vi "Feed Module (Main).vi"(7 "Name of Parent Panel":string="Main.vi", 9 "New Center Coords":T1={"Horizontal"=470, "Vertical"=200}, 10 "Config":variant, 11 "Main UI Message Queue":refnum<queue>) -> ()   [LabVIEW 2018, in "Feed Module.lvlib"]
doc: "This Continuous Measurement sample project is based on the Queued Message Handler template.\n\nThe Event Handling Loop generates messages based on user interface actions.\n\nThe Message Handling Loop processes messages generated by the Event Handling Loop, or by other messages. There are also Acquisition and Logging message handling loop subVIs, and a chart updating loop."
uses:
  Feed Module.lvlib
  support/Message Queue/Message Cluster.ctl
  <vilib>/Utility/miscctls.llb/LVPoint32TypeDef.ctl
  controls/UI Data.ctl
  controls/UI State.ctl
  Controls/Feed Module Config Cluster.ctl
  Controls/Feed Module Settings Cluster.ctl
  Ismatec ISM 831C/Controls/Ismatech ISM831C Settings Cluster.ctl
  Masterflex 7550-30/Controls/Settings Cluster.ctl
  Mettler Toledo/Controls/Settings Cluster.ctl
  Bronkhorst M13 Flow Meter/Settings Cluster.ctl
  Measure Instrument/PID 2 Parameters Cluster.ctl
  Measure Instrument/PID Input Enum.ctl
  Measure Instrument/PID 2 Output Enum.ctl
  Tacmina QI/Tacmina QI DAQ Setting.ctl
  KNF Pump/Settings Cluster plus SIMDOS.ctl
  ASIA Pump/Pump Settings.ctl
  VICI M50 Party Mode/Settings Cluster.ctl
  FLOM Pump/Settings Cluster.ctl
  SSI PR Class/SSI PR or LD Settings Cluster.ctl
  Masterflex 75211/Masterflex 75211 DAQ Setting.ctl
  SSI PR Class/SSI P40 Settings Cluster.ctl
  Ismatec 78001/Ismatec 4083.ctl
  Bronkhorst M14 Flow Meter/Settings Cluster.ctl
  Controls/Feed Module State Cluster.ctl
  Controls/Feed Module Shared Variable Cluster.ctl
  Controls/Feed Module Display.ctl
  Sequencing/Squence Update Cluster.ctl
  support/Message Queue/Enqueue Message (Single).vi
  support/User Event - Stop/User Event - Stop.lvlib
  support/Support Library.lvlib
  support/Message Queue/Message Queue.lvlib
  Measure Instrument/Feed Module Engine.lvlib
  Bronkhorst M13 Flow Meter/Bronkhorst M13 Flow Meter.lvlib
  Mettler Toledo/Mettler Toledo.lvlib
  Masterflex 7550-30/Masterflex 7550-30.lvlib
  Ismatec ISM 831C/Ismatec ISM 831C.lvlib
  Operation Window.vi
  Tacmina QI/Tacmina QI.lvlib
  KNF Pump/KNF SIMDOS.lvlib
  ASIA Pump.lvlib
  Sequencing/Sequencing Library.lvlib
  VICI M50 Party Mode/VICI M6 M50 Party Mode.lvlib
  FLOM Pump/FLOM Pump.lvlib
  support/Command Log VIs/Command Logging.lvlib
  SSI PR Class/SSI PR or LD Pump.lvlib
  Masterflex 75211/Masterflex 75211.lvlib
  SSI PR Class/SSI P40 Pump.lvlib
  Ismatec 78001/Ismatec 4308.lvlib
  Bronkhorst M14 Flow Meter/Bronkhorst M14 Flow Meter.lvlib
panel:
  out "Pump On?":enum16{"Off", "On", "Not Initialized"}(ring)
  out "Pump Flow":dbl
  out "PSIG":dbl format="%#_4g"
  in  "Operation Window":bool
  out "Flow":dbl caption="g/min" format="%.2f"
  out "Ring":u16(ring)=2
  out "Log File path":path
  out "Status":string
  in  "Exit":bool
  out "kg/m^3":dbl format="%#1_4g"
  out "g":dbl format="%#_4g"
  out "C":dbl format="%#_4g"
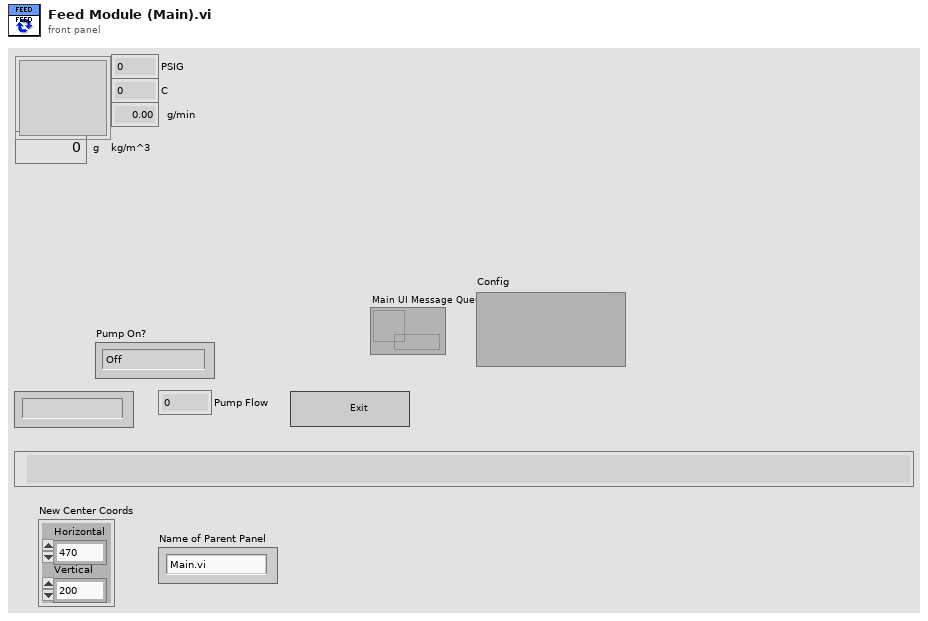
[diagram p1: front panel]
types:
  T1 = typedef "LVPoint32TypeDef.ctl" = cluster{"Horizontal":i32, "Vertical":i32}
  T2 = enum32{"Invalid", "Default", "Floating", "Floating/Auto-Hide", "Modal"}
  T3 = typedef "Feed Module.lvlib/Feed Module State Cluster.ctl" = cluster{"Shared Variables":T4, "Feed Module Config":T5}
  T4 = typedef "Feed Module.lvlib/Feed Module Shared Variable Cluster.ctl" = cluster{"PID 1 Process Variable":string, "PID 1 Output":string, "PID 1 Setpoint":string, "PID 1 Setpoint SV refnum":refnum<k21>, "PID 1 Process Variable SV refnum":refnum<k21>, "PID 1 Output SV refnum":refnum<k21>}
  T5 = typedef "Feed Module.lvlib/Feed Module Config Cluster.ctl" = cluster{"GUID":string, "Drop Coords":T1, "Process Name":string, "Queue Name":string, "Settings":T6, "Settings Load Count":i32, "OP Load Count":i32}
  T6 = typedef "Feed Module.lvlib/Feed Module Settings Cluster.ctl" = cluster{"Cycle Period":dbl, "Ismatech":T7, "Masterflex":T8, "Mettler":T9, "Bronkhorst M13 Flow Meter":T10, "PID 2 Parameters":T11, "Manual Entry":dbl, "Auto?":bool, "output range":cluster{"output high":dbl, "output low":dbl}, "Tacmina Settings":T14, "KNF SIMDOS Settings":T15, "ASIA Pump C":T16, "VICI Settings":T17, "FLOM Settings":T18, "SSI PR/LD Settings":T19, "Masterflex 75211 Settings":T20, "SSI P40 Settings":T21, "Ismatech 3 Channel Settings":T22, "Bronkhorst M14 Settings":T23}
  T7 = typedef "Ismatec ISM 831C.lvlib/Ismatech ISM831C Settings Cluster.ctl" = cluster{"VISA resource name":refnum<visa-resource-name>, "Simulated?":bool, "Pump Number":dbl, "Reverse?":bool}
  T8 = typedef "Masterflex 7550-30.lvlib/Settings Cluster.ctl" = cluster{"VISA resource name":refnum<visa-resource-name>, "Simulated?":bool, "Pump Number":dbl, "Reverse?":bool}
  T9 = typedef "Mettler Toledo.lvlib/Settings Cluster.ctl" = cluster{"VISA resource name":refnum<visa-resource-name>, "Simulated?":bool}
  T10 = typedef "Bronkhorst M13 Flow Meter.lvlib/Settings Cluster.ctl" = cluster{"VISA resource name":refnum<visa-resource-name>, "Simulated?":bool, "Smoothing Steps":i32}
  T11 = typedef "PID 2 Parameters Cluster.ctl" = cluster{"Input Device":T12, "Output Device":T13, "Setpoint":dbl, "PID gains":cluster{"proportional gain (Kc)":dbl, "integral time (Ti, min)":dbl, "derivative time (Td, min)":dbl}}
  T12 = typedef "PID Input Enum.ctl" = enum16{"Default", "Bronkhorst M13", "Bronkhorst M14", "Scale Rate of Change"}
  T13 = typedef "PID 2 Output Enum.ctl" = enum16{"Default", "Ismatec ISM 4308", "Ismatec ISM 831C", "Masterflex 7550-30", "VICI", "Tacmina QI", "KNF SIMDOS", "ASIA Type C", "FLOM UI-22-11", "SSI PR/LD", "SSI P40", "Masterflex 75211-70"}
  T14 = typedef "Tacmina QI.lvlib/Tacmina QI DAQ Setting.ctl" = cluster{"Analog DAQ Task":refnum<k21>, "Digital DAQ Task":refnum<k21>}
  T15 = typedef "KNF SIMDOS.lvlib/Settings Cluster plus SIMDOS.ctl" = cluster{"VISA resource name":refnum<visa-resource-name>, "Simulated?":bool}
  T16 = typedef "ASIA Pump.lvlib/Pump Settings.ctl" = cluster{"ASIA Pump #":i32, "channel":i32, "Simulated":bool}
  T17 = typedef "VICI M6 M50 Party Mode.lvlib/Settings Cluster.ctl" = cluster{"VISA resource name":refnum<visa-resource-name>, "Simulated?":bool, "Pump Letter":string, "Reverse?":bool}
  T18 = typedef "FLOM Pump.lvlib/Settings Cluster.ctl" = cluster{"VISA resource name":refnum<visa-resource-name>, "Simulated?":bool, "Pump Number":dbl}
  T19 = typedef "SSI PR or LD Pump.lvlib/SSI PR or LD Settings Cluster.ctl" = cluster{"VISA resource name":refnum<visa-resource-name>, "Simulated?":bool}
  T20 = typedef "Masterflex 75211.lvlib/Masterflex 75211 DAQ Setting.ctl" = cluster{"Analog DAQ Task":refnum<k21>, "Digital DAQ Task":refnum<k21>}
  T21 = typedef "SSI P40 Pump.lvlib/SSI P40 Settings Cluster.ctl" = cluster{"VISA resource name":refnum<visa-resource-name>, "Simulated?":bool}
  T22 = typedef "Ismatec 4308.lvlib/Ismatec 4083.ctl" = cluster{"VISA resource name":refnum<visa-resource-name>, "Pump Number":i16, "Channel Number":i16, "Simulated?":bool, "Reverse?":bool}
  T23 = typedef "Bronkhorst M14 Flow Meter.lvlib/Settings Cluster.ctl" = cluster{"VISA resource name":refnum<visa-resource-name>, "Simulated?":bool, "Smoothing Steps":i32}
  T24 = typedef "UI State.ctl" = enum16{"Idle", "Acquiring and Logging", "Waiting for Exit", "Waiting for Exit (Acq Stopped)", "Waiting for Exit (Log Stopped)", "Waiting for Stop", "Waiting for Stop (Acq Stopped)", "Waiting for Stop (Log Stopped)"}
  T25 = typedef "UI Data.ctl" = cluster{"Start Ref":refnum<vi>, "Trigger Ref":refnum<vi>, "Stop Ref":refnum<vi>, "Settings Ref":refnum<vi>, "Status Ref":refnum<vi>, "Exit Ref":refnum<vi>, "Data Ref":refnum<vi>}
  T26 = typedef "Feed Module.lvlib/Feed Message Queues.ctl" = cluster{"UI":refnum<queue>, "Engine":refnum<queue>, "FM Display":refnum<queue>, "OP Display":refnum<queue>}
  T27 = typedef "Feed Module.lvlib/Feed Module Display.ctl" = cluster{"Flow":dbl, "Density":dbl, "FL Temp":dbl, "Scale Value":dbl, "Pump On?":enum16{"Off", "On", "Not Initialized"}, "Cycle Period":dbl, "Input Device":T12, "Output":T13, "Pump's Pressure":dbl, "Pump's Flow ":dbl}
  T28 = cluster{"Shift":bool, "Ctrl":bool, "Alt":bool, "Cmd":bool, "Opt":bool}
  T29 = typedef "Sequencing Library.lvlib/Squence Update Cluster.ctl" = cluster{"Auto?":bool, "Manual Entry":dbl, "Setpoint":dbl}
  T30 = enum8{"Enabled", "Disabled", "Disabled and Grayed Out"}
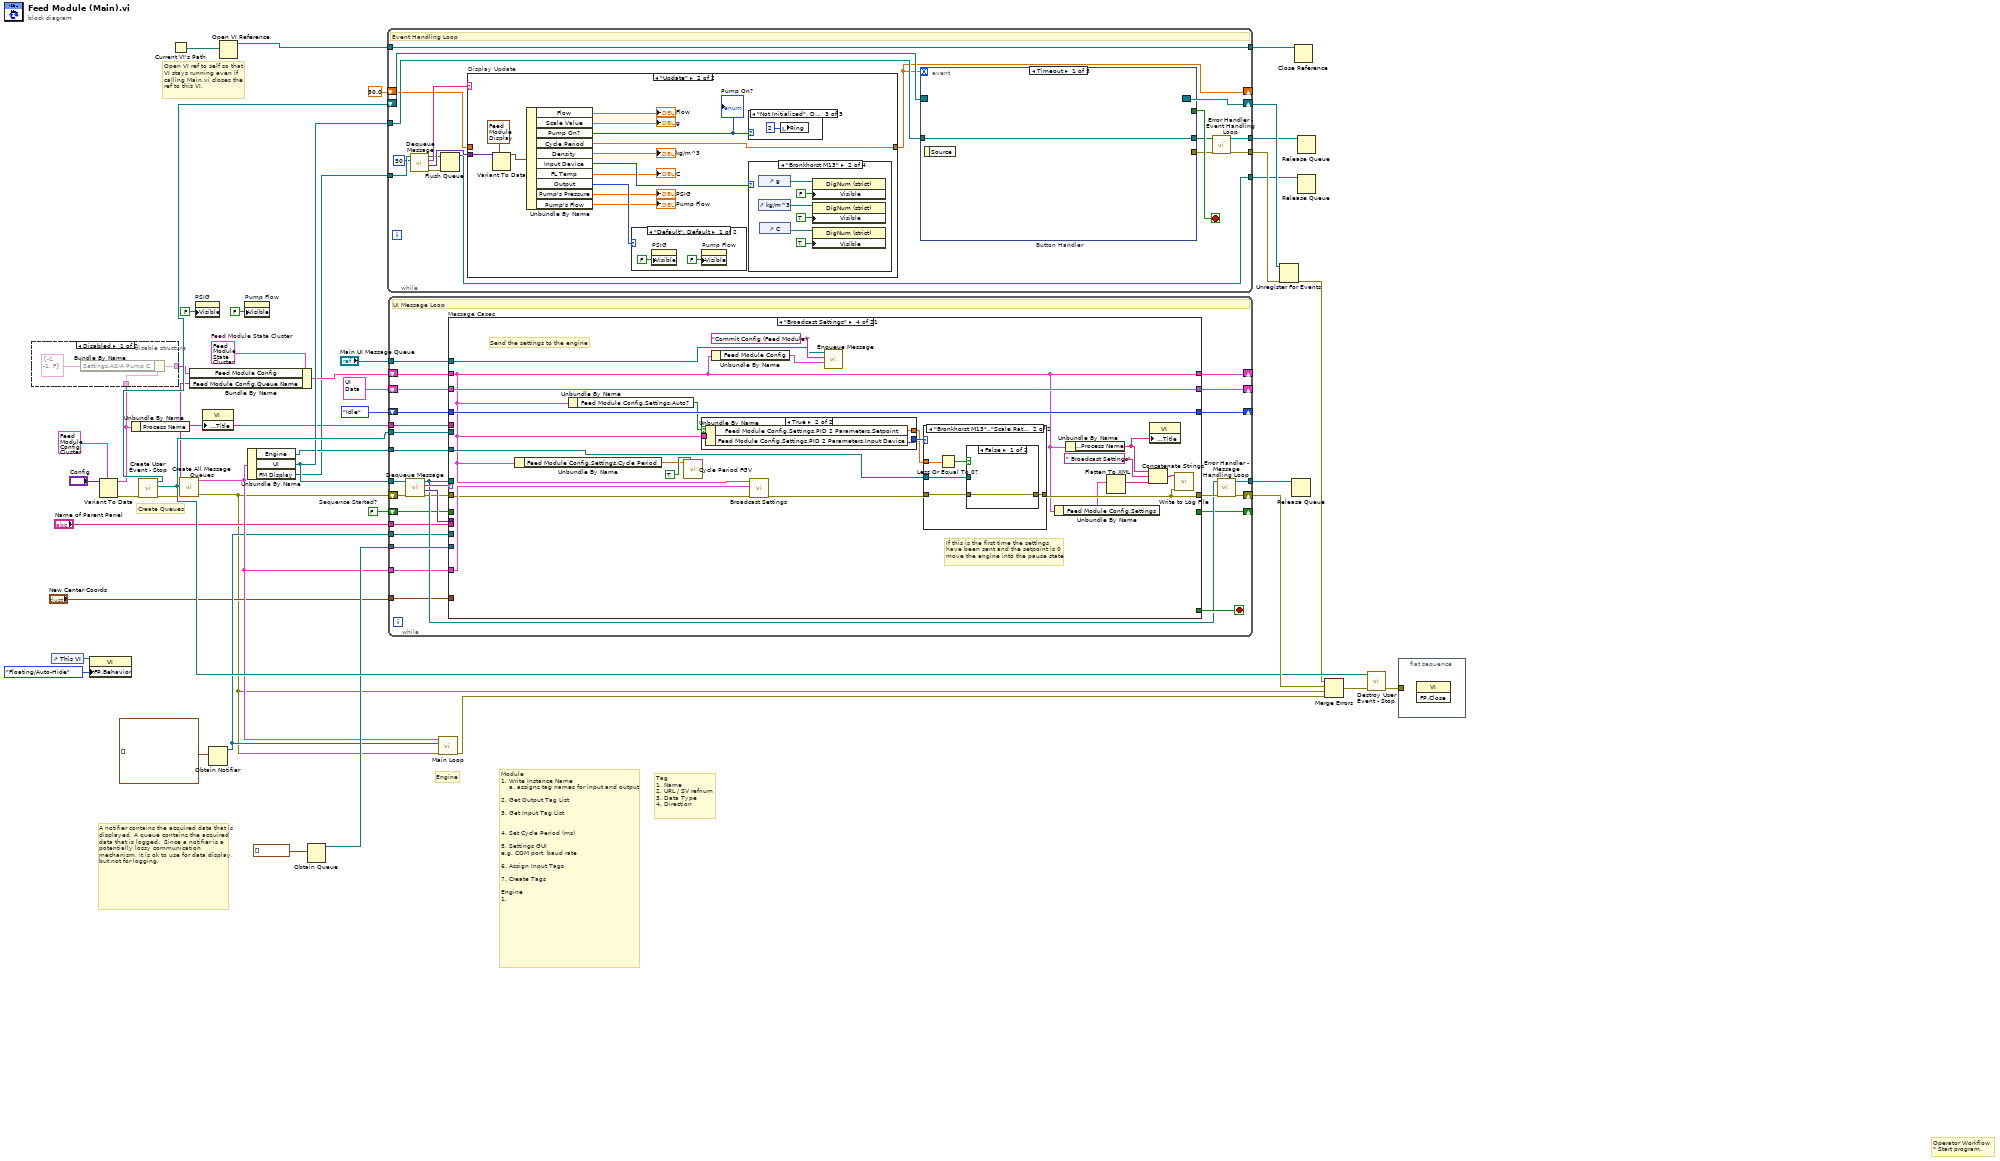
[diagram p0: block diagram]
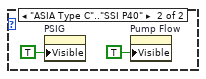
[diagram p4: hidden frame]
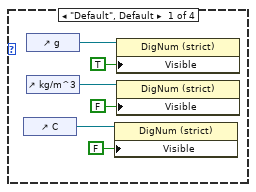
[diagram p5: hidden frame]
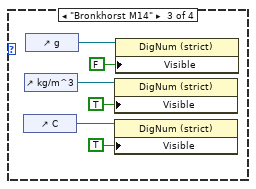
[diagram p6: hidden frame]
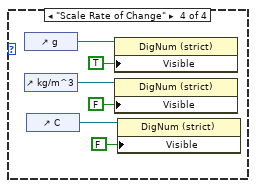
[diagram p7: hidden frame]
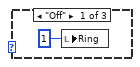
[diagram p8: hidden frame]
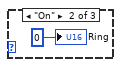
[diagram p9: hidden frame]
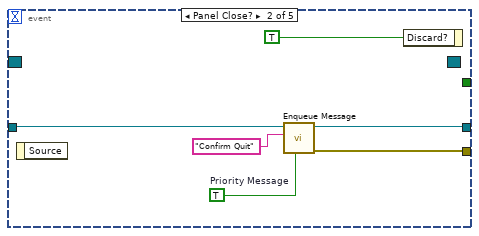
[diagram p10: hidden frame]
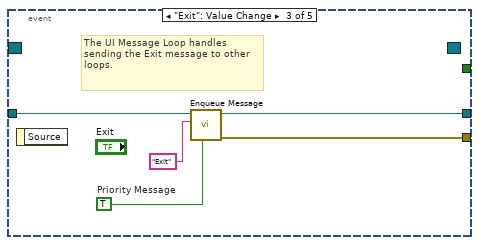
[diagram p11: hidden frame]
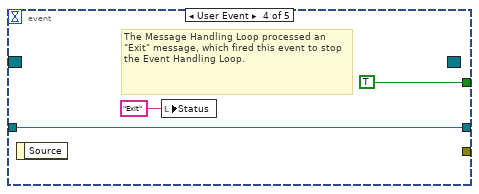
[diagram p12: hidden frame]
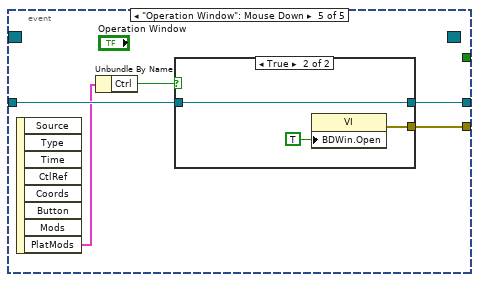
[diagram p13: hidden frame]
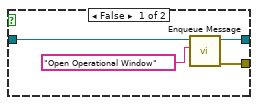
[diagram p14: hidden frame]
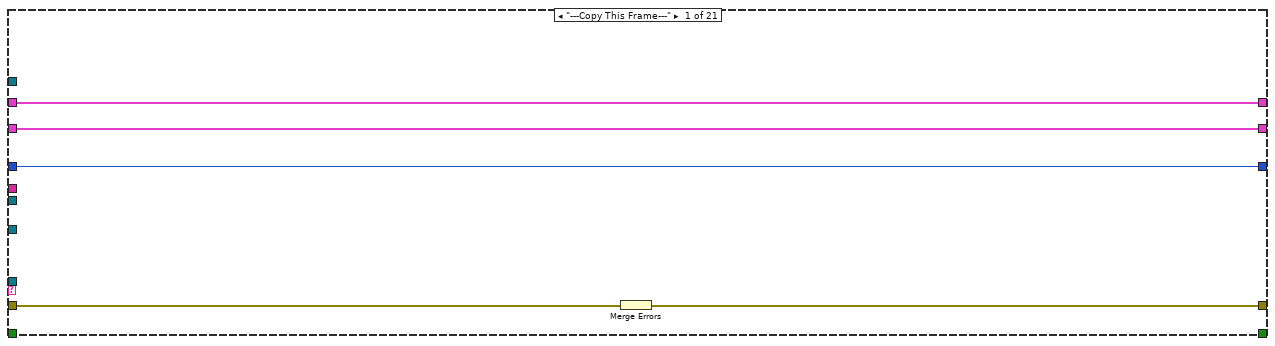
[diagram p15: hidden frame]
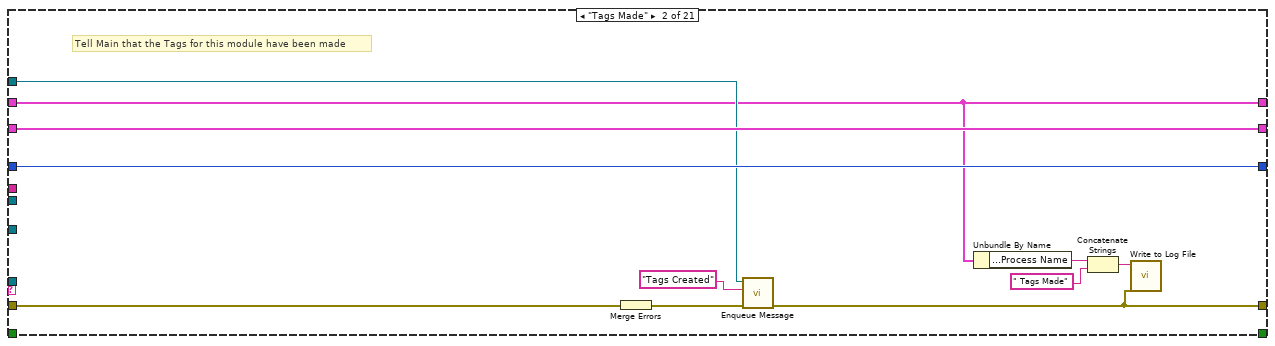
[diagram p16: hidden frame]
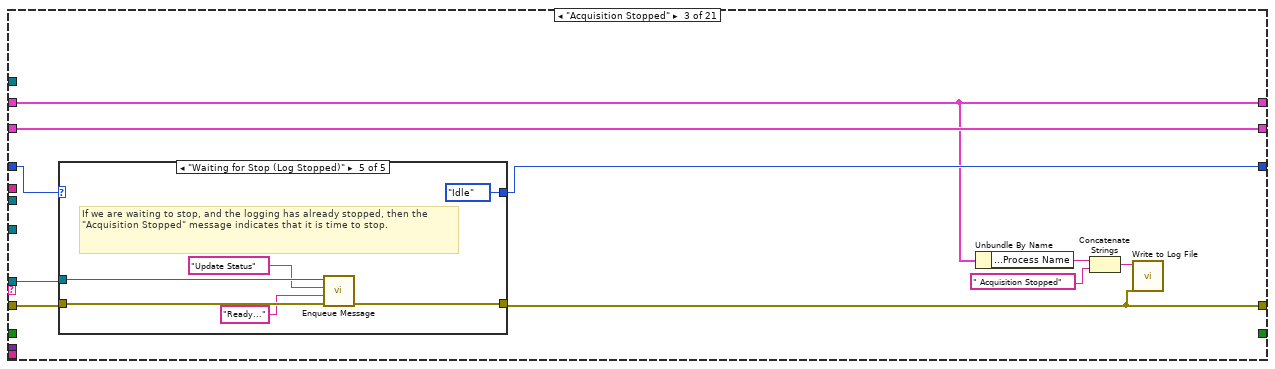
[diagram p17: hidden frame]
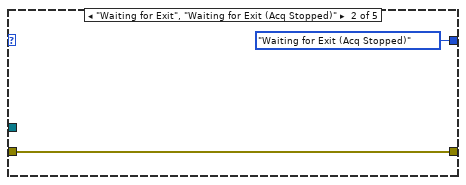
[diagram p19: hidden frame]
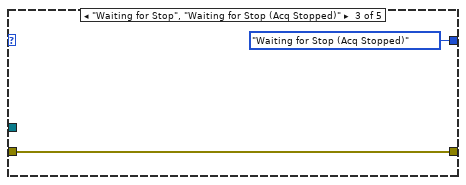
[diagram p20: hidden frame]
diagram:
  w13 = FALSE  # Sequence Started?
  w18 = T3 {"Shared Variables"={"PID 1 Process Variable"="PID1-Mettler Toledo Scale 1", "PID 1 Output"="PID1-Mettler Toledo Scale 1", "PID 1 Setpoint"="PID1-Setpoint", "PID 1 Setpoint SV refnum"="ni.var.psp://localhost/Flow Module 1/PID1-Setpoint", "PID 1 Process Variable SV refnum"="ni.var.psp://localhost/Flow Module 1/PID1-Setpoint", "PID 1 Output SV refnum"="ni.var.psp://localhost/Flow Module 1/PID1-Setpoint"}, "Feed Module Config"={"GUID"="", "Drop Coords"={"Horizontal"=0, "Vertical"=0}, "Process Name"="", "Queue Name"="", "Settings"={"Cycle Period"=500.0, "Ismatech"={"VISA resource name"="", "Simulated?"=TRUE, "Pump Number"=1.0, "Reverse?"=FALSE}, "Masterflex"={"VISA resource name"="", "Simulated?"=TRUE, "Pump Number"=1.0, "Reverse?"=FALSE}, "Mettler"={"VISA resource name"="", "Simulated?"=FALSE}, "Bronkhorst M13 Flow Meter"={"VISA resource name"="", "Simulated?"=TRUE, "Smoothing Steps"=1}, "PID 2 Parameters"={"Input Device"=enum."Default", "Output Device"=enum."Default", "Setpoint"=0.0, "PID gains"={"proportional gain (Kc)"=1.0, "integral time (Ti, min)"=0.01, "derivative time (Td, min)"=0.0}}, "Manual Entry"=0.0, "Auto?"=TRUE, "output range"={"output high"=100.0, "output low"=0.0}, "Tacmina Settings"={"Analog DAQ Task"="", "Digital DAQ Task"=""}, "KNF SIMDOS Settings"={"VISA resource name"="", "Simulated?"=TRUE}, "ASIA Pump C"={"ASIA Pump #"=0, "channel"=0, "Simulated"=FALSE}, "VICI Settings"={"VISA resource name"="", "Simulated?"=TRUE, "Pump Letter"="", "Reverse?"=FALSE}, "FLOM Settings"={"VISA resource name"="", "Simulated?"=TRUE, "Pump Number"=0.0}, "SSI PR/LD Settings"={"VISA resource name"="", "Simulated?"=FALSE}, "Masterflex 75211 Settings"={"Analog DAQ Task"="", "Digital DAQ Task"=""}, "SSI P40 Settings"={"VISA resource name"="", "Simulated?"=TRUE}, "Ismatech 3 Channel Settings"={"VISA resource name"="", "Pump Number"=1, "Channel Number"=0, "Simulated?"=TRUE, "Reverse?"=FALSE}, "Bronkhorst M14 Settings"={"VISA resource name"="", "Simulated?"=FALSE, "Smoothing Steps"=1}}, "Settings Load Count"=0, "OP Load Count"=0}}  # Feed Module State Cluster
  # "Create Queues"
  # "Open VI ref to self so that\nVI stays running even if\ncalling Main.vi closes the\nref to this VI."
  # "Engine"
  # "Operator Workflow\n* Start program."
  # "Module \n1. Write Instance Name\n    a. assigns tag names for input and output\n\n2. Get Output Tag List\n\n3. Get Input Tag List\n\n\n4. Set Cycle Period (ms)\n\n5. Settings GUI\ne.g. COM port, baud rate\n\n6. Assign Input Tags\n\n7. Create Tags\n\nEngine\n1."
  # "Tag\n1. Name\n2. URL / SV refnum\n3. Data Type\n4. Direction"
  # "A notifier contains the acquired data that is displayed. A queue contains the acquired data that is logged.  Since a notifier is a potentially lossy communication mechanism, it is ok to use for data display, but not for logging."
  n1 = control-ref of="This VI"() -> (w2:refnum<vi>)
  n2 = property class="VI"(reference=w2, "FP.Behavior"=T2."Floating/Auto-Hide" ("Front Panel Window:Behavior")) -> ()  [unwired: 1 in, 2 out]
  n3 = Variant To Data(type=T5 {"GUID"="", "Drop Coords"={"Horizontal"=0, "Vertical"=0}, "Process Name"="", "Queue Name"="", "Settings"={"Cycle Period"=500.0, "Ismatech"={"VISA resource name"="", "Simulated?"=TRUE, "Pump Number"=1.0, "Reverse?"=FALSE}, "Masterflex"={"VISA resource name"="", "Simulated?"=TRUE, "Pump Number"=1.0, "Reverse?"=FALSE}, "Mettler"={"VISA resource name"="", "Simulated?"=FALSE}, "Bronkhorst M13 Flow Meter"={"VISA resource name"="", "Simulated?"=TRUE, "Smoothing Steps"=1}, "PID 2 Parameters"={"Input Device"=enum."Default", "Output Device"=enum."Default", "Setpoint"=0.0, "PID gains"={"proportional gain (Kc)"=1.0, "integral time (Ti, min)"=0.01, "derivative time (Td, min)"=0.0}}, "Manual Entry"=0.0, "Auto?"=TRUE, "output range"={"output high"=100.0, "output low"=0.0}, "Tacmina Settings"={"Analog DAQ Task"="", "Digital DAQ Task"=""}, "KNF SIMDOS Settings"={"VISA resource name"="", "Simulated?"=TRUE}, "ASIA Pump C"={"ASIA Pump #"=0, "channel"=0, "Simulated"=FALSE}, "VICI Settings"={"VISA resource name"="", "Simulated?"=TRUE, "Pump Letter"="", "Reverse?"=FALSE}, "FLOM Settings"={"VISA resource name"="", "Simulated?"=TRUE, "Pump Number"=0.0}, "SSI PR/LD Settings"={"VISA resource name"="", "Simulated?"=FALSE}, "Masterflex 75211 Settings"={"Analog DAQ Task"="", "Digital DAQ Task"=""}, "SSI P40 Settings"={"VISA resource name"="", "Simulated?"=TRUE}, "Ismatech 3 Channel Settings"={"VISA resource name"="", "Pump Number"=1, "Channel Number"=0, "Simulated?"=TRUE, "Reverse?"=FALSE}, "Bronkhorst M14 Settings"={"VISA resource name"="", "Simulated?"=FALSE, "Smoothing Steps"=1}}, "Settings Load Count"=0, "OP Load Count"=0} ("Feed Module Config"), Variant="Config") -> (data=w9:T5, error out=w21:errorcluster)  [unwired: 1 in]
  n4 = disable-structure shown="Disabled" {
    disable-tunnel: w9 -> [w46 w48]
    disable-tunnel: [w45 w48] -> w8
    frame Disabled {
      n5 = Bundle By Name(cluster=w46, "Settings.ASIA Pump C"=T16 {"ASIA Pump #"=-1, "channel"=-1, "Simulated"=FALSE}) -> (w45:T5)
    }
    frame Enabled {
    }
  }
  n6 = Unbundle By Name(w9) -> ("Process Name"=w7:string)
  n7 = call "Create User Event - Stop.vi"("error in (no error)"=w21) -> ("error out"=w39:errorcluster, "User Event - Stop"=w40:refnum<user-event>, "Stop Event Registration Refnum"=w41:refnum<event-registration>)  [unwired: 8 in]
  n8 = Current VI's Path() -> (path=w24:path)
  n9 = call "Create All Message Queues.vi"("error in (no error)"=w39, "Process Name"=w7) -> ("error out"=w12:errorcluster, "Message Queues"=w28:T26)  [unwired: 8 in]
  n10 = Bundle By Name(cluster=w18, "Feed Module Config"=w8, "Feed Module Config.Queue Name"=w7) -> (w22:T3)
  n11 = property on="PSIG" class="DigNum (strict)"("Visible"=FALSE) -> ()  [unwired: 2 in, 2 out]
  n12 = property class="VI"("Front Panel.Title"=w7) -> ()  [unwired: 2 in, 2 out]
  n13 = Obtain Notifier(notification data type=waveform(dbl)[] []) -> (notifier out=w27:refnum<notifier>)  [unwired: 3 in, 2 out]
  n14 = Open VI Reference(vi path=w24) -> (vi reference=w25:refnum<vi>)  [unwired: 5 in, 1 out]
  n15 = property on="Pump Flow" class="DigNum (strict)"("Visible"=FALSE) -> ()  [unwired: 2 in, 2 out]
  n16 = Unbundle By Name(w28) -> ("Engine"=w31:refnum<queue>, "UI"=w35:refnum<queue>, "FM Display"=w17:refnum<queue>)
  n17 = Obtain Queue(element data type=waveform(dbl)[] []) -> (queue out=w30:refnum<queue>)  [unwired: 4 in, 2 out]
  n18 = while {
    tunnel: w35 -> [w60]
    tunnel: [w62] -> w43
    shift-right: [w61] -> w37
    shift-left: w41 -> [w66]
    tunnel: [w59] -> w26
    tunnel: w25 -> [w59]
    tunnel: w17 -> [w58]
    shift-right: [w55] -> _
    shift-left: 50.0 ("Cycle Period") -> [w54]
    tunnel: [w50] -> w5
    tunnel: [w49] -> w4
    stop <- w65 stop-if-true
    # "Event Handling Loop"
    n19 = call "Dequeue Message.vi"("timeout in ms (-1)"=50, "Message Queue"=w58) -> ("error out"=w51:errorcluster, "Message Data"=w56:variant, "Message"=w57:string, "dup Message Queue"=w52:refnum<queue>)  [unwired: 6 in]
    n20 = Flush Queue(queue=w52, error in (no error)=w51) -> (queue out=w49:refnum<queue>)  [unwired: 2 out]
    n21 = case "Display Update" shown="\"Update\"" w57 {
      tunnel: w56 -> [_ w80]
      tunnel: [w67 w74] -> w55
      tunnel: w54 -> [w67 _]
      frame "False", Default {
      }
      frame "Update" {
        n22 = Variant To Data(type=T27 {"Flow"=0.0, "Density"=0.0, "FL Temp"=0.0, "Scale Value"=0.0, "Pump On?"=enum."Off", "Cycle Period"=500.0, "Input Device"=enum."Bronkhorst M13", "Output"=enum."Default", "Pump's Pressure"=0.0, "Pump's Flow "=0.0}, Variant=w80) -> (data=w78:T27)  [unwired: 1 in, 1 out]
        n23 = Unbundle By Name(w78) -> ("Flow"=→"Flow":dbl, "Scale Value"=→"g":dbl, "Pump On?"=w75:enum16{"Off", "On", "Not Initialized"}, "Cycle Period"=w74:dbl, "Density"=→"kg/m^3":dbl, "Input Device"=w73:T12, "FL Temp"=→"C":dbl, "Output"=w70:T13, "Pump's Pressure"=→"PSIG":dbl, "Pump's Flow"=→"Pump Flow":dbl)
        "Pump On?" <- w75
        n24 = case shown="\"Default\", Default" w70 {
          frame "Default", Default {
            n25 = property on="PSIG" class="DigNum (strict)"("Visible"=FALSE) -> ()  [unwired: 2 in, 2 out]
            n26 = property on="Pump Flow" class="DigNum (strict)"("Visible"=FALSE) -> ()  [unwired: 2 in, 2 out]
          }
          frame "ASIA Type C".."SSI P40" {
            n27 = property on="PSIG" class="DigNum (strict)"("Visible"=TRUE) -> ()  [unwired: 2 in, 2 out]
            n28 = property on="Pump Flow" class="DigNum (strict)"("Visible"=TRUE) -> ()  [unwired: 2 in, 2 out]
          }
        }
        n29 = case shown="\"Not Initialized\", Default" w75 {
          frame "Off" {
            n30 = local write "Ring"(u16 1 ("Ring")) -> ()
          }
          frame "On" {
            "Ring" <- u16 0 ("Ring")
          }
          frame "Not Initialized", Default {
            n31 = local write "Ring"(u16 2 ("Ring")) -> ()
          }
        }
        n32 = case shown="\"Bronkhorst M13\"" w73 {
          frame "Default", Default {
            n33 = control-ref of="C"() -> (w86:refnum<vi>)
            n34 = control-ref of="g"() -> (w89:refnum<vi>)
            n35 = control-ref of="kg/m^3"() -> (w90:refnum<vi>)
            n36 = property class="DigNum (strict)"(reference=w86, "Visible"=FALSE) -> ()  [unwired: 1 in, 2 out]
            n37 = property class="DigNum (strict)"(reference=w89, "Visible"=TRUE) -> ()  [unwired: 1 in, 2 out]
            n38 = property class="DigNum (strict)"(reference=w90, "Visible"=FALSE) -> ()  [unwired: 1 in, 2 out]
          }
          frame "Bronkhorst M13" {
            n39 = control-ref of="g"() -> (w95:refnum<vi>)
            n40 = control-ref of="kg/m^3"() -> (w96:refnum<vi>)
            n41 = control-ref of="C"() -> (w92:refnum<vi>)
            n42 = property class="DigNum (strict)"(reference=w95, "Visible"=FALSE) -> ()  [unwired: 1 in, 2 out]
            n43 = property class="DigNum (strict)"(reference=w96, "Visible"=TRUE) -> ()  [unwired: 1 in, 2 out]
            n44 = property class="DigNum (strict)"(reference=w92, "Visible"=TRUE) -> ()  [unwired: 1 in, 2 out]
          }
          frame "Bronkhorst M14" {
            n45 = control-ref of="C"() -> (w97:refnum<vi>)
            n46 = control-ref of="kg/m^3"() -> (w102:refnum<vi>)
            n47 = control-ref of="g"() -> (w101:refnum<vi>)
            n48 = property class="DigNum (strict)"(reference=w102, "Visible"=TRUE) -> ()  [unwired: 1 in, 2 out]
            n49 = property class="DigNum (strict)"(reference=w97, "Visible"=TRUE) -> ()  [unwired: 1 in, 2 out]
            n50 = property class="DigNum (strict)"(reference=w101, "Visible"=FALSE) -> ()  [unwired: 1 in, 2 out]
          }
          frame "Scale Rate of Change" {
            n51 = control-ref of="g"() -> (w107:refnum<vi>)
            n52 = control-ref of="kg/m^3"() -> (w108:refnum<vi>)
            n53 = control-ref of="C"() -> (w103:refnum<vi>)
            n54 = property class="DigNum (strict)"(reference=w107, "Visible"=TRUE) -> ()  [unwired: 1 in, 2 out]
            n55 = property class="DigNum (strict)"(reference=w108, "Visible"=FALSE) -> ()  [unwired: 1 in, 2 out]
            n56 = property class="DigNum (strict)"(reference=w103, "Visible"=FALSE) -> ()  [unwired: 1 in, 2 out]
          }
        }
      }
    }
    n57 = event "Button Handler" shown="[0] Timeout" {
      selector: w66 -> [_ _ _ _ _]
      dyn-events: [_ _ _ _ _] -> w61
      timeout: w55 -> [_ _ _ _ _]
      tunnel: [_ _ _ TRUE ("Discard?") _] -> w65
      tunnel: w60 -> [w112 w115 w120 w124 w129]
      tunnel: [_ w113 w123 _ w131] -> w63
      tunnel: [w112 w114 w119 w124 w130] -> w64
      event Timeout {
        n58 = event-data() -> ()  [unwired: 1 in, 1 out]
      }
      event Panel Close? {
        w116 = TRUE  # Priority Message
        n59 = event-data() -> ()  [unwired: 1 in, 1 out]
        n60 = call-poly "Enqueue Message.vi"("Priority Message? (F)"=w116, "Message"="Confirm Quit", "Message Queue"=w115) -> ("error out"=w113:errorcluster, "dup Message Queue"=w114:refnum<queue>)  [unwired: 7 in]
        n61 = event-data("Discard?"=TRUE) -> ()  [unwired: 1 in, 1 out]
      }
      event "Exit": Value Change {
        w121 = TRUE  # Priority Message
        # "The UI Message Loop handles sending the Exit message to other loops."
        n62 = event-data() -> ()  [unwired: 1 in, 1 out]
        n63 = call-poly "Enqueue Message.vi"("Priority Message? (F)"=w121, "Message"="Exit", "Message Queue"=w120) -> ("error out"=w123:errorcluster, "dup Message Queue"=w119:refnum<queue>)  [unwired: 7 in]
      }
      event User Event {
        # "The Message Handling Loop processed an \"Exit\" message, which fired this event to stop the Event Handling Loop."
        n64 = event-data() -> ()  [unwired: 1 in, 1 out]
        n65 = local write "Status"("Exit" ("Exit String")) -> ()
      }
      event "Operation Window": Mouse Down {
        n66 = event-data() -> ("PlatMods"=w128:T28)  [unwired: 1 in, 7 out]
        n67 = Unbundle By Name(w128) -> ("Ctrl"=w127:bool)
        n68 = case shown="True" w127 {
          tunnel: [w135 w136] -> w131
          tunnel: [w134 w137] -> w130
          tunnel: w129 -> [w133 w137]
          frame False {
            n69 = call-poly "Enqueue Message.vi"("Message"="Open Operational Window", "Message Queue"=w133) -> ("error out"=w135:errorcluster, "dup Message Queue"=w134:refnum<queue>)  [unwired: 8 in]
          }
          frame True {
            n70 = property class="VI"("BDWin.Open"=TRUE ("Block Diagram Window:Open")) -> (error out=w136:errorcluster)  [unwired: 2 in, 1 out]
          }
        }
      }
    }
    n71 = call "Error Handler - Event Handling Loop.vi"("error in (no error)"=w63, "Message Queue"=w64) -> ("dup error in"=w62:errorcluster, "dup Message Queue"=w50:refnum<queue>)  [unwired: 8 in]
  }
  n72 = while {
    tunnel: w35 -> [w160]
    tunnel: w40 -> [w164]
    shift-right: [w154] -> w44
    shift-left: w12 -> [w163]
    shift-right: [w159] -> _
    shift-left: w22 -> [w142]
    shift-right: [w157] -> _
    shift-left: T25 {"Start Ref"=refnum, "Trigger Ref"=refnum, "Stop Ref"=refnum, "Settings Ref"=refnum, "Status Ref"=refnum, "Exit Ref"=refnum, "Data Ref"=refnum} ("Measurement UI Controls") -> [w158]
    tunnel: w27 -> [w144]
    tunnel: w30 -> [w156]
    shift-right: [w152] -> _
    shift-left: UI_State."Idle" ("UI State") -> [w146]
    tunnel: w31 -> [w151]
    tunnel: w28 -> [w143]
    tunnel: "Main UI Message Queue" -> [w147]
    tunnel: "Name of Parent Panel" -> [w150]
    tunnel: w7 -> [w149]
    tunnel: "New Center Coords" -> [w148]
    shift-right: [w140] -> _
    shift-left: w13 -> [w141]
    tunnel: [w139] -> w3
    stop <- w165 stop-if-true
    # "UI Message Loop"
    n73 = call "Dequeue Message.vi"("error in (no error)"=w163, "Message Queue"=w160) -> ("error out"=w145:errorcluster, "Message Data"=w161:variant, "Message"=w162:string, "dup Message Queue"=w153:refnum<queue>)  [unwired: 6 in]
    n74 = case "Message Cases" shown="\"Broadcast Settings\"" w162 {
      selector: w162 -> [_ _ _ _ _ _ _ _ _ _ _ _ _ _ _ _ _ _ _ _ w595]
      tunnel: w153 -> [_ _ w187 _ w255 _ w311 w327 w358 w383 _ w421 w439 w453 _ w501 _ _ w572 _ _]
      tunnel: w145 -> [w170 w181 w188 w225 w254 w280 w296 w326 w362 w387 w406 w416 _ w454 w485 w499 w518 w532 w557 w589 _]
      tunnel: [w169 w172 w183 w217 w249 w281 w288 w315 w347 w365 w406 w408 w431 w449 w481 w493 w520 w534 w549 w576 w596] -> w155
      tunnel: [_ _ _ _ _ _ _ _ _ TRUE _ _ _ _ _ _ _ _ _ _ _] -> w165
      tunnel: w161 -> [_ _ _ _ _ w283 _ _ w361 w371 _ _ w437 _ _ _ _ _ _ w588 _]
      tunnel: w164 -> [_ _ _ _ _ _ _ _ _ w386 _ _ _ _ _ _ _ _ _ _ _]
      tunnel: [w168 w171 w182 w211 w248 w286 w287 w314 w349 w364 w405 w407 w429 w448 w480 w492 w519 w533 w548 w575 w601] -> w159
      tunnel: w158 -> [w167 w180 w191 w230 w257 w285 w308 w324 w363 w384 w404 w417 w441 w457 w489 w516 w525 w542 w569 w585 w606]
      tunnel: [w167 w180 w191 w230 w257 w285 w308 w324 w363 w384 w403 w417 w441 w457 w489 w516 w525 w542 w569 w585 w606] -> w157
      tunnel: w156 -> [_ _ _ _ _ _ _ _ _ w378 _ _ _ _ _ _ _ _ _ _ _]
      tunnel: w146 -> [w166 w179 w190 w229 w256 w279 w297 _ w353 _ _ _ w440 w456 w477 _ _ _ w558 w580 w605]
      tunnel: [w166 w179 w189 w229 w253 w279 w298 UI_State."Acquiring and Logging" ("UI State") w353 UI_State."Idle" ("UI State") UI_State."Idle" ("UI State") UI_State."Idle" ("UI State") w440 w455 w477 UI_State."Acquiring and Logging" ("UI State") UI_State."Acquiring and Logging" ("UI State") UI_State."Acquiring and Logging" ("UI State") w559 w580 w605] -> w152
      tunnel: w151 -> [_ _ _ w224 _ _ w295 _ _ w376 _ _ _ _ _ _ w523 w540 w556 _ _]
      tunnel: w150 -> [_ _ _ _ _ _ _ _ _ _ _ w415 _ _ _ _ _ _ _ _ _]
      tunnel: w149 -> [_ _ _ _ _ _ _ _ _ _ _ w412 _ _ _ _ _ _ _ _ _]
      tunnel: w148 -> [_ _ _ _ _ _ _ _ _ _ _ w414 _ _ _ _ _ _ _ _ _]
      tunnel: w147 -> [_ w177 _ w210 _ _ _ _ _ w369 _ _ _ _ w488 _ _ _ _ _ _]
      tunnel: w144 -> [_ _ _ _ _ _ _ _ _ w382 _ _ _ _ w487 _ _ _ _ _ _]
      tunnel: w143 -> [_ _ _ w228 _ _ _ _ _ _ _ _ _ _ w486 _ _ _ _ _ _]
      tunnel: w142 -> [w168 w171 w182 w211 w248 w286 w287 w314 w349 w364 w405 w407 w430 w448 w479 w492 w519 w533 w548 w575 w601]
      tunnel: w141 -> [_ _ _ _ _ _ _ w323 _ _ _ _ _ _ _ _ _ _ _ _ _]
      tunnel: [_ _ _ _ _ _ _ w320 _ _ _ _ _ _ _ _ _ _ _ _ _] -> w140
      frame "---Copy This Frame---" {
        # "Duplicate this frame when creating new messages.  Change this comment in the duplicated frame to describe this message."
        n75 = Merge Errors(w170) -> (w169:errorcluster)
      }
      frame "Tags Made" {
        # "Tell Main that the Tags for this module have been made"
        # "Duplicate this frame when creating new messages.  Change this comment in the duplicated frame to describe this message."
        n76 = Merge Errors(w181) -> (w176:errorcluster)
        n77 = call-poly "Enqueue Message.vi"("error in (no error)"=w176, "Message"="Tags Created", "Message Queue"=w177) -> ("error out"=w172:errorcluster)  [unwired: 7 in, 1 out]
        n78 = Unbundle By Name(w171) -> ("Feed Module Config.Process Name"=w175:string)
        n79 = Concatenate Strings(w175, " Tags Made" ("text")) -> (w173:string)
        n80 = call "Write to Log File.vi"("error in"=w172, "text"=w173) -> ()  [unwired: 9 in, 1 out]
      }
      frame "Acquisition Stopped" {
        # "Logic for determining what action to take when the acquisition has stopped."
        n81 = case shown="\"Waiting for Stop (Log Stopped)\"" w190 {
          selector: w190 -> [w193 _ _ _ _]
          tunnel: [w193 UI_State."Waiting for Exit (Acq Stopped)" ("UI State") UI_State."Waiting for Stop (Acq Stopped)" ("UI State") UI_State."Idle" ("UI State") UI_State."Idle" ("UI State")] -> w189
          tunnel: w188 -> [w192 w194 w196 w202 w208]
          tunnel: [w192 w194 w196 w201 w207] -> w183
          tunnel: w187 -> [_ _ _ w200 w206]
          frame Default {
          }
          frame "Waiting for Exit", "Waiting for Exit (Acq Stopped)" {
          }
          frame "Waiting for Stop", "Waiting for Stop (Acq Stopped)" {
          }
          frame "Waiting for Exit (Log Stopped)" {
            # "If we are waiting to exit, and the logging has already stopped, then the \"Acquisition Stopped\" message indicates that it is time to exit."
            n82 = call-poly "Enqueue Message.vi"("Priority Message? (F)"=TRUE, "error in (no error)"=w202, "Message"="Exit", "Message Queue"=w200) -> ("error out"=w201:errorcluster)  [unwired: 6 in, 1 out]
          }
          frame "Waiting for Stop (Log Stopped)" {
            # "If we are waiting to stop, and the logging has already stopped, then the \"Acquisition Stopped\" message indicates that it is time to stop."
            n83 = call-poly "Enqueue Message.vi"("error in (no error)"=w208, "Message Data"="Ready..." ("Message"), "Message"="Update Status", "Message Queue"=w206) -> ("error out"=w207:errorcluster)  [unwired: 6 in, 1 out]
          }
        }
        n84 = Unbundle By Name(w182) -> ("Feed Module Config.Process Name"=w186:string)
        n85 = Concatenate Strings(w186, " Acquisition Stopped" ("text")) -> (w184:string)
        n86 = call "Write to Log File.vi"("error in"=w183, "text"=w184) -> ()  [unwired: 9 in, 1 out]
      }
      frame "Broadcast Settings" {
        # "If this is the first time the settings\nhave been sent and the setpoint is 0 \nmove the engine into the pause state"
        # "Send the settings to the engine"
        # "Send the 'Update Settings' message to the Logging and Acquisition message loops."
        n87 = Unbundle By Name(w211) -> ("Feed Module Config.Settings.Cycle Period"=w226:dbl)
        n88 = Unbundle By Name(w211) -> ("Feed Module Config.Settings.Auto?"=w220:bool)
        n89 = call "Cycle Period FGV.vi"("Write"=TRUE, "Cycle Period In (ms)"=w226) -> ()  [unwired: 8 in, 2 out]
        n90 = case shown="True" w220 {
          tunnel: [w231 w236] -> w222
          tunnel: [w232 w235] -> w221
          tunnel: w211 -> [w233 w234]
          frame False {
            n91 = Unbundle By Name(w233) -> ("Feed Module Config.Settings.Manual Entry"=w232:dbl, "Feed Module Config.Settings.PID 2 Parameters.Input Device"=w231:T12)
          }
          frame True {
            n92 = Unbundle By Name(w234) -> ("Feed Module Config.Settings.PID 2 Parameters.Setpoint"=w235:dbl, "Feed Module Config.Settings.PID 2 Parameters.Input Device"=w236:T12)
          }
        }
        n93 = Unbundle By Name(w211) -> ("Feed Module Config"=w213:T5)
        n94 = call "Broadcast Settings.vi"("error in (no error)"=w225, "Message Queues"=w228, "Feed Module State Cluster in"=w211) -> ("error out"=w223:errorcluster)  [unwired: 8 in]
        n95 = call-poly "Enqueue Message.vi"("Message Data"=w213, "Message"="Commit Config (Feed Module)", "Message Queue"=w210) -> ()  [unwired: 7 in, 2 out]
        n96 = case shown="\"Bronkhorst M13\"..\"Scale Rate of Change\"" w222 {
          tunnel: w223 -> [w237 w242]
          tunnel: w224 -> [_ w241]
          tunnel: [w237 w240] -> w217
          tunnel: w221 -> [_ w239]
          frame "Default", Default {
          }
          frame "Bronkhorst M13".."Scale Rate of Change" {
            n97 = Less Or Equal To 0?(x=w239) -> (x <= 0?=w238:bool)
            n98 = case shown="False" w238 {
              tunnel: w242 -> [w243 w247]
              tunnel: w241 -> [_ w246]
              tunnel: [w243 w245] -> w240
              frame False {
              }
              frame True {
                n99 = call-poly "Enqueue Message.vi"("error in (no error)"=w247, "Message"="Pause", "Message Queue"=w246) -> ("error out"=w245:errorcluster)  [unwired: 7 in, 1 out]
              }
            }
          }
        }
        n100 = Unbundle By Name(w211) -> ("Feed Module Config.Settings"=w216:T6)
        n101 = Unbundle By Name(w211) -> ("Feed Module Config.Process Name"=w214:string)
        n102 = Flatten To XML(anything=w216) -> (xml string=w215:string)
        n103 = Concatenate Strings(w214, " Broadcast Settings" ("text"), w215) -> (w218:string)
        n104 = property class="VI"("Front Panel.Title"=w214) -> ()  [unwired: 2 in, 2 out]
        n105 = call "Write to Log File.vi"("error in"=w217, "text"=w218) -> ()  [unwired: 9 in, 1 out]
      }
      frame "Confirm Quit" {
        # "Confirm Quit - Message that can confirm whether or not the user wants to exit the application."
        n106 = case shown="\"Acquiring and Logging\"" w256 {
          tunnel: w255 -> [w262 w268]
          tunnel: w254 -> [w261 w266]
          tunnel: [w258 w265] -> w249
          tunnel: [UI_State."Idle" ("UI State") w264] -> w253
          frame Default {
            # "If 'Confirm Quit' comes in while the system is idle, there is no need for a confirmation message."
            n107 = call-poly "Enqueue Message.vi"("Priority Message? (F)"=TRUE, "error in (no error)"=w261, "Message"="Exit", "Message Queue"=w262) -> ("error out"=w258:errorcluster)  [unwired: 6 in, 1 out]
          }
          frame "Acquiring and Logging" {
            n108 = Two Button Dialog(message="Are you sure you want to quit while the acquisition is running?" ("Confirm Quit Message"), 1:"No" ("No"), 2:"Yes" ("Yes")) -> (T button?=w267:bool)
            n109 = case shown="True" w267 {
              tunnel: w268 -> [_ w278]
              tunnel: w266 -> [w272 w277]
              tunnel: [w272 w276] -> w265
              tunnel: [UI_State."Acquiring and Logging" ("UI State") UI_State."Waiting for Exit" ("UI State")] -> w264
              frame False {
                # "User did not want to quit."
              }
              frame True {
                n110 = call-poly "Enqueue Message.vi"("error in (no error)"=w277, "Message"="Stop", "Message Queue"=w278) -> ("error out"=w276:errorcluster)  [unwired: 7 in, 1 out]
              }
            }
          }
        }
        n111 = Unbundle By Name(w248) -> ("Feed Module Config.Process Name"=w252:string)
        n112 = Concatenate Strings(w252, " Quit" ("text")) -> (w250:string)
        n113 = call "Write to Log File.vi"("error in"=w249, "text"=w250) -> ()  [unwired: 9 in, 1 out]
      }
      frame "Display Log File Path" {
        n114 = Variant To Data(error in=w280, type=path "", Variant=w283) -> (data=→"Log File path":path, error out=w281:errorcluster)
      }
      frame "E-Stop" {
        # "E-Stop pauses the engine"
        # "Message Acquisition and Logging loops to stop"
        # "Enable: Start, Exit, Settings\nDisable: Stop"
        # "Stop the pumps."
        n115 = Unbundle By Name(w308) -> ("Trigger Ref"=w299:refnum<vi>, "Stop Ref"=w300:refnum<vi>, "Start Ref"=w303:refnum<vi>, "Exit Ref"=w302:refnum<vi>, "Settings Ref"=w301:refnum<vi>)
        n116 = call-poly "Enqueue Message.vi"("error in (no error)"=w296, "Message Data"="Ready..." ("Ready..."), "Message"="Update Status", "Message Queue"=w311) -> ("error out"=w293:errorcluster)  [unwired: 6 in, 1 out]
        n117 = Build Array(w303, w302, w301) -> (w306:refnum<vi>[])
        n118 = Build Array(w299, w300) -> (w305:refnum<vi>[])
        n119 = call-poly "Enqueue Message.vi"("error in (no error)"=w293, "Message"="Pause", "Message Queue"=w295) -> ("error out"=w292:errorcluster)  [unwired: 7 in, 1 out]
        n120 = call "Set Enable State on Multiple Controls.vi"("Enable?"=FALSE, "Controls"=w305) -> ()  [unwired: 10 in]
        n121 = call "Set Enable State on Multiple Controls.vi"("Enable?"=TRUE, "Controls"=w306) -> ()  [unwired: 10 in]
        n122 = case shown="Default" w297 {
          selector: w297 -> [_ w313]
          tunnel: [UI_State."Waiting for Stop" ("UI State") w313] -> w298
          frame Default {
          }
          frame "Waiting for Exit" {
          }
        }
        n123 = Merge Errors(w292) -> (w288:errorcluster)
        n124 = Unbundle By Name(w287) -> ("Feed Module Config.Process Name"=w291:string)
        n125 = Concatenate Strings(w291, " E-STOP" ("text")) -> (w289:string)
        n126 = call "Write to Log File.vi"("error in"=w288, "text"=w289) -> ()  [unwired: 9 in, 1 out]
      }
      frame "Sequence Start" {
        # "Clear chart"
        # "Message Acquisition and Logging loops to start"
        # "Enable: Stop\nDisable: Start, Exit, Settings"
        # "Stop the pumps."
        n127 = Unbundle By Name(w324) -> ("Trigger Ref"=w331:refnum<vi>, "Stop Ref"=w332:refnum<vi>, "Start Ref"=w335:refnum<vi>, "Exit Ref"=w334:refnum<vi>, "Settings Ref"=w333:refnum<vi>, "Data Ref"=w329:refnum<vi>)
        n128 = property class="WFChart (strict)"(reference=w329, "History Data"=waveform(dbl)[][] []) -> ()  [unwired: 1 in, 2 out]
        n129 = Build Array(w335, w334, w333) -> (w338:refnum<vi>[])
        n130 = Build Array(w331, w332) -> (w337:refnum<vi>[])
        n131 = call-poly "Enqueue Message.vi"("error in (no error)"=w326, "Message"="Broadcast settings", "Message Queue"=w327) -> ("error out"=w321:errorcluster, "dup Message Queue"=w322:refnum<queue>)  [unwired: 7 in]
        n132 = call "Set Enable State on Multiple Controls.vi"("Enable?"=TRUE, "Controls"=w337) -> ()  [unwired: 10 in]
        n133 = call "Set Enable State on Multiple Controls.vi"("Enable?"=FALSE, "Controls"=w338) -> ()  [unwired: 10 in]
        n134 = case shown="False" w323 {
          selector: w323 -> [_ w345]
          tunnel: [w344 w345] -> w320
          tunnel: w321 -> [w343 w346]
          tunnel: w322 -> [w341 _]
          tunnel: [w340 w346] -> w319
          frame False {
            w344 = TRUE  # Sequence Started?
            n135 = call-poly "Enqueue Message.vi"("error in (no error)"=w343, "Message"="Start Loops", "Message Queue"=w341) -> ("error out"=w340:errorcluster)  [unwired: 7 in, 1 out]
          }
          frame True {
          }
        }
        n136 = Merge Errors(w319) -> (w315:errorcluster)
        n137 = Unbundle By Name(w314) -> ("Feed Module Config.Process Name"=w318:string)
        n138 = Concatenate Strings(w318, " Sequence Start" ("text")) -> (w316:string)
        n139 = call "Write to Log File.vi"("error in"=w315, "text"=w316) -> ()  [unwired: 9 in, 1 out]
      }
      frame "Error" {
        # "Stop if there is an error"
        # "Error - Check the error message data and respond accordingly. This message is sent by the \"Error Handler\" VIs at the end of each loop in this application."
        n140 = Variant To Data(error in=w362, type=errorcluster {"status"=FALSE, "code"=0, "source"=""} ("error out"), Variant=w361) -> (data=w359:errorcluster, error out=w355:errorcluster)
        n141 = call <vilib>:"General Error Handler.vi"("error in (no error)"=w359) -> ("message"=w348:string)  [unwired: 10 in, 4 out]
        n142 = call-poly "Enqueue Message.vi"("Priority Message? (F)"=TRUE, "Message"="Exit", "Message Queue"=w358) -> ("error out"=w354:errorcluster)  [unwired: 7 in, 1 out]
        n143 = Merge Errors(w354, w355) -> (w347:errorcluster)
        n144 = Unbundle By Name(w349) -> ("Feed Module Config.Process Name"=w352:string)
        n145 = Concatenate Strings(w352, " Error: " ("text"), w348) -> (w350:string)
        n146 = call "Write to Log File.vi"("error in"=w347, "text"=w350) -> ()  [unwired: 9 in, 1 out]
      }
      frame "Exit" {
        w373 = TRUE  # Delete Module?
        # "Don't check the error outs. The acquisition and logging queues may have already been released."
        # "Close references owned by the Main VI."
        # "Stop the VI"
        # "Exit - Fire the User Event to stop the Event Handling Loop.  Also send Exit messages to the Acquisition and Logging loops."
        n147 = Release Queue(queue=w383, error in (no error)=w387) -> (error out=w381:errorcluster)  [unwired: 1 in, 2 out]
        n148 = call "Fire User Event - Stop.vi"("User Event - Stop"=w386) -> ("error out"=w385:errorcluster)  [unwired: 10 in]
        n149 = Release Notifier(notifier=w382, error in (no error)=w381) -> (error out=w380:errorcluster)  [unwired: 1 in, 2 out]
        n150 = Variant To Data(type=w373, Variant=w371) -> (data=w372:bool, error out=w374:errorcluster)  [unwired: 1 in]
        n151 = Build Array(w376) -> (w375:refnum<queue>[])
        n152 = Release Queue(queue=w378, error in (no error)=w380) -> (error out=w379:errorcluster)  [unwired: 1 in, 2 out]
        n153 = Select(t=w373, s=w374, f=w372) -> (s? t:f=w370:bool)
        n154 = for {
          tunnel: w375 -> [w394] mode=indexing
          # "Send the engine the stop, exit"
          n155 = call-poly "Enqueue Message.vi"("Message"="Stop", "Message Queue"=w394) -> ("dup Message Queue"=w395:refnum<queue>)  [unwired: 8 in, 1 out]
          n156 = call-poly "Enqueue Message.vi"("Message"="Exit", "Message Queue"=w395) -> ()  [unwired: 8 in, 2 out]
        }
        n157 = case "Don't enqueue Delete Module if opening campaign because it\nwill already have been deleted and new config loaded and we create\na race condition." shown="True" w370 {
          tunnel: w364 -> [_ w391]
          tunnel: w369 -> [_ w389]
          frame False {
          }
          frame True {
            n158 = Unbundle By Name(w391) -> ("Feed Module Config.GUID"=w390:string)
            n159 = call-poly "Enqueue Message.vi"("Message Data"=w390, "Message"="Delete Module", "Message Queue"=w389) -> ()  [unwired: 7 in, 2 out]
          }
        }
        n160 = Merge Errors(w385, w379) -> (w365:errorcluster)
        n161 = Unbundle By Name(w364) -> ("Feed Module Config.Process Name"=w368:string)
        n162 = Concatenate Strings(w368, " Exit" ("text")) -> (w366:string)
        n163 = call "Write to Log File.vi"("error in"=w365, "text"=w366) -> ()  [unwired: 9 in, 1 out]
      }
      frame "Init UI Refs" {
        # "Enable: Start, Exit, Settings\nDisable: Stop"
        # "Init UI Refs - Store control references for UI controls.  Also enable/disable controls appropriately."
        n164 = property class="VI"("Front Panel.Closeable"=TRUE ("Front Panel Window:Closeable")) -> ()  [unwired: 2 in, 2 out]
        n165 = control-ref of="Status"() -> (w401:refnum<vi>)
        n166 = control-ref of="Exit"() -> (w398:refnum<vi>)
        n167 = Bundle By Name(cluster=w404, "Status Ref"=w401, "Exit Ref"=w398) -> (w403:T25)
        n168 = Build Array(w398) -> (w400:refnum<vi>[])
        n169 = call "Set Enable State on Multiple Controls.vi"("Enable?"=TRUE, "Controls"=w400) -> ()  [unwired: 10 in]
      }
      frame "Initialize" {
        # "Initialize - Get configuration settings, then message the UI to initialize, and broadcast the settings to the other message loops."
        n170 = property class="VI" props=["FP.State"]() -> (reference out=w413:refnum<vi>)  [unwired: 2 in, 2 out]
        n171 = call-poly "Enqueue Message.vi"("error in (no error)"=w416, "Message"="Init UI Refs", "Message Queue"=w421) -> ("error out"=w419:errorcluster, "dup Message Queue"=w420:refnum<queue>)  [unwired: 7 in]
        n172 = call-poly "Enqueue Message.vi"("error in (no error)"=w419, "Message"="Broadcast Settings", "Message Queue"=w420) -> ("error out"=w427:errorcluster, "dup Message Queue"=w426:refnum<queue>)  [unwired: 7 in]
        n173 = call "Make Child and Move.vi"("Process Name"=w412, "Name of Parent Panel"=w415, "New Center Coords"=w414, "VI in"=w413) -> ()  [unwired: 8 in]
        n174 = call-poly "Enqueue Message.vi"("error in (no error)"=w427, "Message Data"="Ready..." ("Ready..."), "Message"="Update Status", "Message Queue"=w426) -> ("error out"=w408:errorcluster)  [unwired: 6 in, 1 out]
        n175 = Unbundle By Name(w407) -> ("Feed Module Config.Process Name"=w411:string)
        n176 = Concatenate Strings(w411, " Initialize" ("text")) -> (w409:string)
        n177 = call "Write to Log File.vi"("error in"=w408, "text"=w409) -> ()  [unwired: 9 in, 1 out]
      }
      frame "Sequence Update" {
        # "#CHECK DISABLE"
        # "Update the Sequence settings from the Sequence Dialog"
        # "Launch the Settings Dialog when the user clicks the 'Settings' button."
        n178 = Variant To Data(type=T29 {"Auto?"=TRUE, "Manual Entry"=0.0, "Setpoint"=0.0} ("Cluster"), Variant=w437) -> (data=w436:T29)  [unwired: 1 in, 1 out]
        n179 = in-place {
          in-place-border: w436 -> [w447]
          n180 = in-place-cluster #1(w430) -> ("Feed Module Config"=w443:T5)
          n181 = Unbundle By Name(w447) -> ("Auto?"=w446:bool, "Manual Entry"=w445:dbl, "Setpoint"=w444:dbl)
          n182 = Bundle By Name(cluster=w443, "Settings.Auto?"=w446, "Settings.Manual Entry"=w445, "Settings.PID 2 Parameters.Setpoint"=w444) -> (w442:T5)
          n183 = in-place-cluster #1("Feed Module Config"=w442) -> (w429:T3)
        }
        n184 = call-poly "Enqueue Message.vi"("Message"="Broadcast Settings", "Message Queue"=w439) -> ("error out"=w435:errorcluster)  [unwired: 8 in, 1 out]
        n185 = Merge Errors(w435) -> (w431:errorcluster)
        n186 = Unbundle By Name(w429) -> ("Feed Module Config.Process Name"=w434:string)
        n187 = Concatenate Strings(w434, " Sequence Update" ("text")) -> (w432:string)
        n188 = call "Write to Log File.vi"("error in"=w431, "text"=w432) -> ()  [unwired: 9 in, 1 out]
      }
      frame "Logging Stopped" {
        # "Logic for determining what action to take when the logging has stopped."
        n189 = case shown="\"Waiting for Stop (Acq Stopped)\"" w456 {
          selector: w456 -> [w459 _ _ _ _]
          tunnel: [w459 UI_State."Waiting for Exit (Log Stopped)" ("UI State") UI_State."Waiting for Stop (Log Stopped)" ("UI State") UI_State."Idle" ("UI State") UI_State."Idle" ("UI State")] -> w455
          tunnel: w454 -> [w458 w460 w462 w468 w474]
          tunnel: [w458 w460 w462 w467 w473] -> w449
          tunnel: w453 -> [_ _ _ w466 w472]
          frame Default {
          }
          frame "Waiting for Exit", "Waiting for Exit (Log Stopped)" {
          }
          frame "Waiting for Stop", "Waiting for Stop (Log Stopped)" {
          }
          frame "Waiting for Exit (Acq Stopped)" {
            # "If we are waiting to exit, and the acquisition has already stopped, then the \"Logging Stopped\" message indicates that it is time to exit."
            n190 = call-poly "Enqueue Message.vi"("Priority Message? (F)"=TRUE, "error in (no error)"=w468, "Message"="Exit", "Message Queue"=w466) -> ("error out"=w467:errorcluster)  [unwired: 6 in, 1 out]
          }
          frame "Waiting for Stop (Acq Stopped)" {
            # "If we are waiting to stop, and the acquisition has already stopped, then the \"Logging Stopped\" message indicates that it is time to stop."
            n191 = call-poly "Enqueue Message.vi"("error in (no error)"=w474, "Message Data"="Ready..." ("Message"), "Message"="Update Status", "Message Queue"=w472) -> ("error out"=w473:errorcluster)  [unwired: 6 in, 1 out]
          }
        }
        n192 = Unbundle By Name(w448) -> ("Feed Module Config.Process Name"=w452:string)
        n193 = Concatenate Strings(w452, " Logging Stopped" ("text")) -> (w450:string)
        n194 = call "Write to Log File.vi"("error in"=w449, "text"=w450) -> ()  [unwired: 9 in, 1 out]
      }
      frame "Open Operational Window" {
        # "Duplicate this frame when creating new messages.  Change this comment in the duplicated frame to describe this message."
        n195 = in-place {
          n196 = in-place-cluster #2(w479) -> ("Feed Module Config.OP Load Count"=w491:i32)
          n197 = Increment(x=w491) -> (x+1=w490:i32)
          n198 = in-place-cluster #2("Feed Module Config.OP Load Count"=w490) -> (w478:T3)
        }
        n199 = local read "Pump On?"() -> (w476:enum16{"Off", "On", "Not Initialized"})
        n200 = call-by-ref "?"("Main UI Message Queue"=w488, "Pump On?"=w476, "error in (no error)"=w485, "Graph Notifier"=w487, "Message Queues"=w486, "Feed Module State Cluster in"=w478) -> ("error out"=w481:errorcluster, "Feed Module State Cluster out"=w480:T3)  [unwired: 5 in, 3 out]
        n201 = Unbundle By Name(w480) -> ("Feed Module Config.Process Name"=w484:string)
        n202 = Concatenate Strings(w484, " Open OP Window" ("text")) -> (w482:string)
        n203 = call "Write to Log File.vi"("error in"=w481, "text"=w482) -> ()  [unwired: 9 in, 1 out]
      }
      frame "Start" {
        # "We only have one loop but i've kept this in anyway"
        # "Clear chart"
        # "Message Acquisition and Logging loops to start"
        # "Enable: Stop\nDisable: Start, Exit, Settings"
        # "Start - Enable/Disable buttons appropriately for an acquisition that has started, and update status display."
        n204 = Unbundle By Name(w516) -> ("Trigger Ref"=w507:refnum<vi>, "Stop Ref"=w508:refnum<vi>, "Start Ref"=w511:refnum<vi>, "Exit Ref"=w510:refnum<vi>, "Settings Ref"=w509:refnum<vi>, "Data Ref"=w498:refnum<vi>)
        n205 = property class="WFChart (strict)"(reference=w498, "History Data"=waveform(dbl)[][] []) -> ()  [unwired: 1 in, 2 out]
        n206 = Build Array(w511, w510, w509) -> (w514:refnum<vi>[])
        n207 = Build Array(w507, w508) -> (w513:refnum<vi>[])
        n208 = call-poly "Enqueue Message.vi"("error in (no error)"=w499, "Message"="Broadcast settings", "Message Queue"=w501) -> ("error out"=w502:errorcluster, "dup Message Queue"=w500:refnum<queue>)  [unwired: 7 in]
        n209 = call "Set Enable State on Multiple Controls.vi"("Enable?"=TRUE, "Controls"=w513) -> ()  [unwired: 10 in]
        n210 = call "Set Enable State on Multiple Controls.vi"("Enable?"=FALSE, "Controls"=w514) -> ()  [unwired: 10 in]
        n211 = call-poly "Enqueue Message.vi"("error in (no error)"=w502, "Message"="Start Loops", "Message Queue"=w500) -> ("error out"=w503:errorcluster)  [unwired: 7 in, 1 out]
        n212 = Merge Errors(w503) -> (w493:errorcluster)
        n213 = Unbundle By Name(w492) -> ("Feed Module Config.Process Name"=w496:string)
        n214 = Concatenate Strings(w496, " Start" ("text")) -> (w494:string)
        n215 = call "Write to Log File.vi"("error in"=w493, "text"=w494) -> ()  [unwired: 9 in, 1 out]
      }
      frame "Start Loops" {
        # "I'm not entirly sure where we would have a second Process Name in a module but i'm leaving it for now"
        # "Message Acquisition and Logging loops to start"
        # "Start - Enable/Disable buttons appropriately for an acquisition that has started, and update status display."
        n216 = Unbundle By Name(w519) -> ("Feed Module Config.Process Name"=w521:string)
        n217 = Build Array(w523) -> (w522:refnum<queue>[])
        n218 = for {
          tunnel: w518 -> [w529]
          tunnel: [w528] -> w517 mode=indexing
          tunnel: w522 -> [w527] mode=indexing
          tunnel: w521 -> [w526]
          n219 = call-poly "Enqueue Message.vi"("error in (no error)"=w529, "Message Data"=w526, "Message"="Start", "Message Queue"=w527) -> ("error out"=w528:errorcluster)  [unwired: 6 in, 1 out]
        }
        n220 = Merge Errors(w518, w517) -> (w520:errorcluster)
      }
      frame "Start Log" {
        # "I'm not entirly sure where we would have a second Process Name in a module but i'm leaving it for now"
        # "Message Acquisition and Logging loops to start"
        # "Start - Enable/Disable buttons appropriately for an acquisition that has started, and update status display."
        n221 = Unbundle By Name(w533) -> ("Feed Module Config.Process Name"=w538:string)
        n222 = Build Array(w540) -> (w539:refnum<queue>[])
        n223 = for {
          tunnel: w532 -> [w546]
          tunnel: [w545] -> w531 mode=indexing
          tunnel: w539 -> [w544] mode=indexing
          tunnel: w538 -> [w543]
          n224 = call-poly "Enqueue Message.vi"("error in (no error)"=w546, "Message Data"=w543, "Message"="Start Log", "Message Queue"=w544) -> ("error out"=w545:errorcluster)  [unwired: 6 in, 1 out]
        }
        n225 = property class="VI"("Front Panel.Title"=w538) -> ()  [unwired: 2 in, 2 out]
        n226 = Merge Errors(w532, w531) -> (w534:errorcluster)
        n227 = Unbundle By Name(w533) -> ("Feed Module Config.Process Name"=w537:string)
        n228 = Concatenate Strings(w537, " Start Log" ("text")) -> (w535:string)
        n229 = call "Write to Log File.vi"("error in"=w534, "text"=w535) -> ()  [unwired: 9 in, 1 out]
      }
      frame "Stop" {
        # "Stop Pauses the engine"
        # "Enable: Start, Exit, Settings\nDisable: Stop"
        # "Stop - Enable/Disable buttons appropriately for an acquisition that has stopped, and update status display."
        n230 = Unbundle By Name(w569) -> ("Trigger Ref"=w560:refnum<vi>, "Stop Ref"=w561:refnum<vi>, "Start Ref"=w564:refnum<vi>, "Exit Ref"=w563:refnum<vi>, "Settings Ref"=w562:refnum<vi>)
        n231 = call-poly "Enqueue Message.vi"("error in (no error)"=w557, "Message Data"="Ready..." ("Ready..."), "Message"="Update Status", "Message Queue"=w572) -> ("error out"=w555:errorcluster)  [unwired: 6 in, 1 out]
        n232 = Build Array(w564, w563, w562) -> (w567:refnum<vi>[])
        n233 = Build Array(w560, w561) -> (w566:refnum<vi>[])
        n234 = call-poly "Enqueue Message.vi"("error in (no error)"=w555, "Message"="Pause", "Message Queue"=w556) -> ("error out"=w553:errorcluster)  [unwired: 7 in, 1 out]
        n235 = call "Set Enable State on Multiple Controls.vi"("Enable?"=FALSE, "Controls"=w566) -> ()  [unwired: 10 in]
        n236 = call "Set Enable State on Multiple Controls.vi"("Enable?"=TRUE, "Controls"=w567) -> ()  [unwired: 10 in]
        n237 = case shown="Default" w558 {
          selector: w558 -> [_ w574]
          tunnel: [UI_State."Waiting for Stop" ("UI State") w574] -> w559
          frame Default {
          }
          frame "Waiting for Exit" {
          }
        }
        n238 = Merge Errors(w553) -> (w549:errorcluster)
        n239 = Unbundle By Name(w548) -> ("Feed Module Config.Process Name"=w552:string)
        n240 = Concatenate Strings(w552, "Stop" ("text")) -> (w550:string)
        n241 = call "Write to Log File.vi"("error in"=w549, "text"=w550) -> ()  [unwired: 9 in, 1 out]
      }
      frame "Update Status" {
        # "Update Display - Convert the message data to a string to display in the Status indicator."
        n242 = Unbundle By Name(w585) -> ("Trigger Ref"=w581:refnum<vi>, "Stop Ref"=w584:refnum<vi>)
        n243 = Variant To Data(error in=w589, type="", Variant=w588) -> (data=w582:string, error out=w586:errorcluster)
        "Status" <- w582
        n244 = property class="Bool"(reference=w584) -> ("DisabledEnum"=w583:T30)  [unwired: 1 in, 2 out]
        n245 = case shown="\"Enabled\"" w583 {
          tunnel: w582 -> [w592 _]
          tunnel: w581 -> [w593 _]
          frame "Enabled" {
            # "Disable the Force Trigger only while we are logging."
            n246 = Build Array(w593) -> (w594:refnum<vi>[])
            n247 = Not Equal?(x="Logging" ("Logging"), y=w592) -> (x != y?=w590:bool)
            n248 = call "Set Enable State on Multiple Controls.vi"("Enable?"=w590, "Controls"=w594) -> ()  [unwired: 10 in]
          }
          frame "Disabled", Default {
          }
        }
        n249 = Merge Errors(w586) -> (w576:errorcluster)
        n250 = Unbundle By Name(w575) -> ("Feed Module Config.Process Name"=w579:string)
        n251 = Concatenate Strings(w579, "Update Status" ("text")) -> (w577:string)
        n252 = call "Write to Log File.vi"("error in"=w576, "text"=w577) -> ()  [unwired: 9 in, 1 out]
      }
      frame Default {
        # "'Default' case only runs if there is a message that isn't defined in any of the other cases.  Output a programming error."
        n253 = Concatenate Strings("The invalid message string " ("string"), w595, " was received in Feed Module Main." ("string")) -> (w597:string)
        n254 = Bundle By Name(cluster=errorcluster {"status"=TRUE, "code"=1, "source"=""} ("error constant"), "source"=w597) -> (w596:errorcluster)
        n255 = Unbundle By Name(w601) -> ("Feed Module Config.Process Name"=w604:string)
        n256 = Concatenate Strings(w604, "Incorrect Message Recieved: " ("text"), w595) -> (w602:string)
        n257 = call "Write to Log File.vi"("error in"=w596, "text"=w602) -> ()  [unwired: 9 in, 1 out]
      }
    }
    n258 = call "Error Handler - Message Handling Loop.vi"("error in (no error)"=w155, "Message Queue"=w153) -> ("dup error in"=w154:errorcluster, "dup Message Queue"=w139:refnum<queue>)  [unwired: 8 in]
  }
  n259 = call "Main Loop.vi"("error in (no error)"=w12, "Chart Notifier"=w27, "Message Queues"=w28) -> ("error out"=w29:errorcluster)  [unwired: 8 in]
  n260 = Unregister For Events(event registration refnum=w37, error in=w43) -> (error out=w38:errorcluster)
  n261 = Release Queue(queue=w3) -> ()  [unwired: 2 in, 3 out]
  n262 = Close Reference(reference=w26) -> ()  [unwired: 1 in, 1 out]
  n263 = Release Queue(queue=w5) -> ()  [unwired: 2 in, 3 out]
  n264 = Release Queue(queue=w4) -> ()  [unwired: 2 in, 3 out]
  n265 = Merge Errors(w38, w44, w12, w29) -> (w42:errorcluster)
  n266 = call "Destroy User Event - Stop.vi"("error in (no error)"=w42, "User Event - Stop"=w40) -> ("error out"=w14:errorcluster)  [unwired: 9 in]
  n267 = flat-sequence {
    tunnel: w14 -> [_]
    frame #0 {
      n268 = invoke class="VI" method="FP.Close"() -> ()  [unwired: 3 in, 3 out]
    }
  }
